vi "Zaber A Series TCPIP Move.vi"() -> ()   [LabVIEW 2015]
doc: "This beginner example shows the Move VI, which allows the user to move devices based on real-world units easily. \n\nThis example is specifically set up to work with Zaber devices accessible over TCP/IP"
uses:
  Zaber A Series.lvlib
panel:
  in  "IP Address":string
  in  "Port Number (7770)":i32=7770
  in  "Units (0: microsteps)":u16(ring) items=["microsteps", "microns", "millimeters", "inches", "degrees"]
  in  "Movement Type (0: relative)":u16(ring) items=["relative", "absolute"]
  in  "Device and Axis":string
  in  "Microstep Size (0)":dbl
  in  "Move Distance (0)":dbl format="%#_6f"
  # "(c) 2017-2021 Zaber Technologies.  ALL RIGHTS RESERVED."
  # "This example shows how you can use the Move VI to make movements easily.\nThe Move VI allows you to use real world units while moving the stage. This is\nuseful because typically you would send movement commands with microstep\nvalues and make conversions to see how it relates to real units. To use these\nunits (except microsteps) make sure to input the Microstep Size before running.\nvalue can be found on spec page for the product on www.zaber.com."
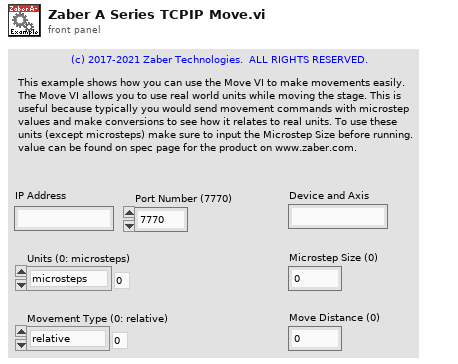
[diagram p1: front panel]
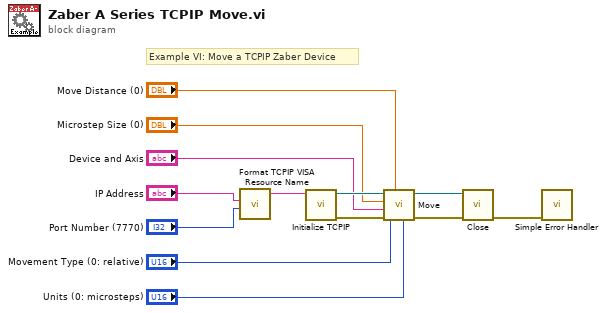
[diagram p0: block diagram]
diagram:
  # "Example VI: Move a TCPIP Zaber Device"
  n1 = call "Format TCPIP VISA Resource Name.vi"("Port Number (7770)"="Port Number (7770)", "Hostname or IP Address"="IP Address") -> ("VISA resource name out"=w3:string)  [unwired: 9 in]
  n2 = call "Initialize TCPIP.vi"("VISA resource name in"=w3) -> ("error out"=w13:errorcluster, "VISA resource name out"=w11:refnum<visa-resource-name>)  [unwired: 9 in]
  n3 = call "Move.vi"("Units (0: microsteps)"="Units (0: microsteps)", "Movement Type (0: relative)"="Movement Type (0: relative)", "Move Distance (0)"="Move Distance (0)", "error in (no error)"=w13, "Device and Axis"="Device and Axis", "Microstep Size (0)"="Microstep Size (0)", "VISA resource name"=w11) -> ("error out"=w4:errorcluster, "VISA resource name out"=w5:refnum<visa-resource-name>)  [unwired: 3 in]
  n4 = call "Close.vi"("error in (no error)"=w4, "VISA resource name"=w5) -> ("error out"=w12:errorcluster)  [unwired: 9 in]
  n5 = call <vilib>:"Simple Error Handler.vi"("error in (no error)"=w12) -> ()  [unwired: 4 in, 5 out]
